vi "Setup Connection Settings.vi"(8 "error in (no error)":errorcluster, 10 "Model in":refnum<class "Model.lvclass">, 11 "Boot Loader in":refnum<class "Boot Loader.lvclass">) -> (0 "error out":errorcluster, 2 "Model out":refnum<class "Model.lvclass">, 3 "Boot Loader out":refnum<class "Boot Loader.lvclass">)   [LabVIEW 2015, in "Boot Loader.lvclass"]
uses:
  Boot Loader.lvclass
  Model/Model.lvclass
  Model/Model.lvclass/Model.ctl
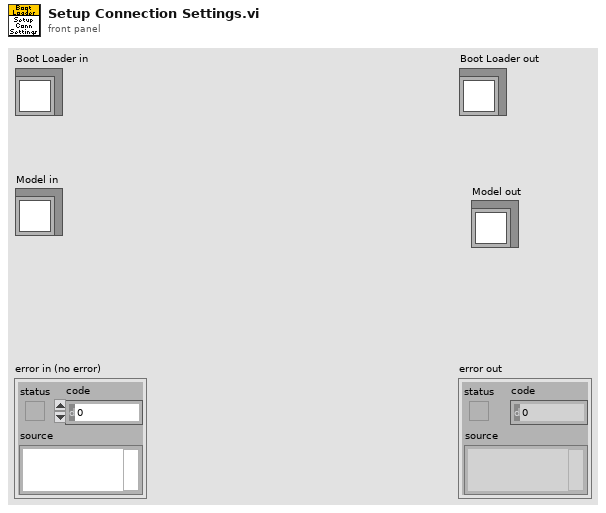
[diagram p1: front panel]
types:
  T1 = typedef "FAMT Typedefs.lvlib/Connection Settings.ctl" = cluster{"Pressure Servo Valve 1 DAC":u8, "Pressure Servo Valve 2 DAC":u8, "Flow Control Valve DAC":u8, "Load Cell ADC":u8, "FC1 ILC Port":refnum<visa-resource-name>, "FC2 ILC Port":refnum<visa-resource-name>, "Tovey A-B Port":refnum<visa-resource-name>, "Tovey C-D Port":refnum<visa-resource-name>, "Tovey E-F Port":refnum<visa-resource-name>, "FC1 ILC Protocol":T2, "FC2 ILC Protocol":T2, "Tovey A-B Protocol":T2, "Tovey C-D Protocol":T2, "Tovey E-F Protocol":T2}
  T2 = typedef "SerialProtocols.lvlib/SerialProtocol.ctl" = enum16{"RS232", "RS485", "SerialSimulator"}
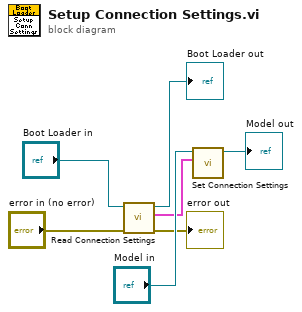
[diagram p0: block diagram]
diagram:
  n1 = call "Read Connection Settings.vi"("error in (no error)"="error in (no error)", "Boot Loader in"="Boot Loader in") -> ("error out"=→"error out":errorcluster, "Connection Settings"=w1:T1, "Boot Loader out"=→"Boot Loader out":refnum<class "Boot Loader.lvclass">)  [unwired: 7 in]
  n2 = call "Set Connection Settings.vi"("Connection Settings"=w1, "Model in"="Model in") -> ("Model out"=→"Model out":refnum<class "Model.lvclass">)  [unwired: 9 in]
